vi "Get Dev Product Type.vi"(8 "error in (no error)":errorcluster, 11 "Refnum in":refnum<k21>) -> (0 "error out":errorcluster, 1 "ProductType":string, 3 "Refnum out":refnum<k21>)   [LabVIEW 2016]
uses:
  <resource>/objmgr/daqmx.rc
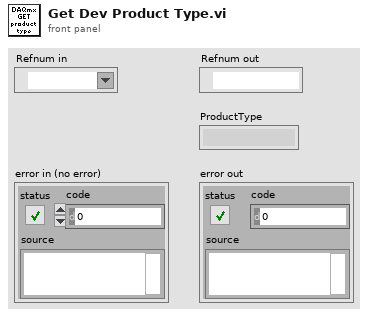
[diagram p1: front panel]
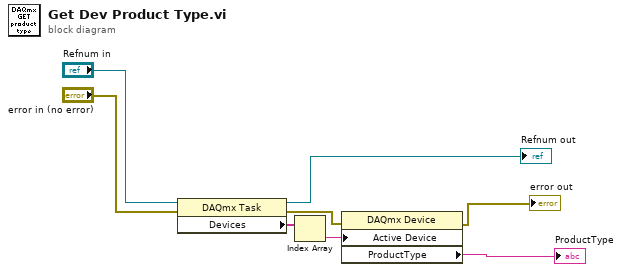
[diagram p0: block diagram]
diagram:
  n1 = property class="DAQmx Task"(reference="Refnum in", error in="error in (no error)") -> (reference out=→"Refnum out":refnum<k21>, error out=w6:errorcluster, "Devices"=w3:tag[])
  n2 = Index Array(array=w3) -> (element=w4:tag)  [unwired: 1 in]
  n3 = property class="DAQmx Device"(error in=w6, "Active Device"=w4) -> (error out=→"error out":errorcluster, "ProductType"=→"ProductType":string)  [unwired: 1 in, 1 out]
